vi "save as.vi"(8 "error in":errorcluster, 11 "state in":T1) -> (0 "error out":errorcluster, 1 "canceled?":bool, 3 "state out":T1)   [LabVIEW 2013, in "RT Temperature Controller.lvlib"]
uses:
  RT Temperature Controller.lvlib
  Controls/StateCluster.ctl
  <vilib>/NI/Tag Bus Data Framework/Configuration Editor/Classes/SystemConfigRepo/SystemConfigRepo.lvclass
  <vilib>/CEF_TreeControl/Node/NodeRef.ctl
  <vilib>/CEF_TreeControl/Node/NISE_CEF_Node.lvclass
  <vilib>/CEF_TreeControl/Node/UserEventRef.ctl
  <vilib>/CEF_TreeControl/Controls/EventCluster.ctl
  SplashScreen/splash screen.ctl
  SplashScreen/notifier data.ctl
  <vilib>/CEF_TreeControl/NISE_CEF_TreeControl.lvlib
  SplashScreen/splash screen.lvlib
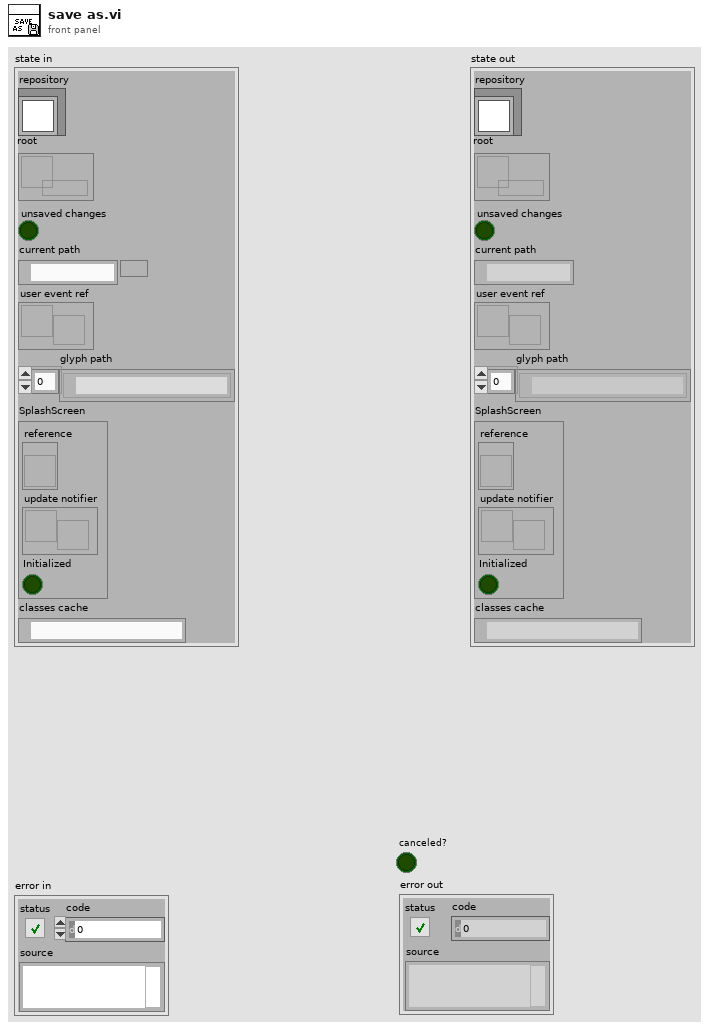
[diagram p1: front panel]
types:
  T1 = typedef "RT Temperature Controller.lvlib/StateCluster.ctl" = cluster{"repository":refnum<class "SystemConfigRepo.lvclass">, "root":T2, "unsaved changes":bool, "current path":path, "user event ref":T3, "glyph path":path[], "SplashScreen":T4, "classes cache":path}
  T2 = typedef "NISE_CEF_Node.lvclass/NodeRef.ctl" = refnum<data-value>
  T3 = typedef "NISE_CEF_Node.lvclass/UserEventRef.ctl" = refnum<user-event>
  T4 = typedef "RT Temperature Controller.lvlib/splash screen.lvlib/splash screen.ctl" = cluster{"reference":refnum<vi>, "update notifier":refnum<notifier>, "Initialized":bool}
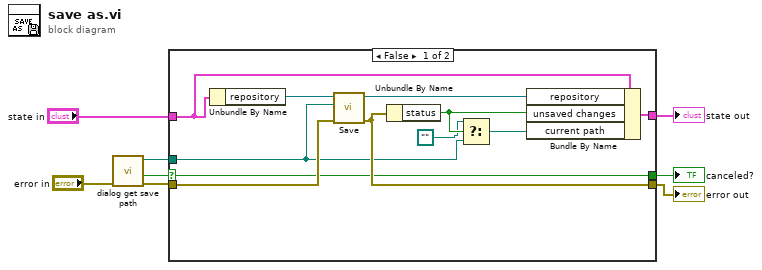
[diagram p0: block diagram]
diagram:
  n1 = call "dialog get save path.vi"("error in"="error in") -> ("error out"=w4:errorcluster, "cancelled"=w2:bool, "selected path"=w3:path)  [unwired: 8 in]
  n2 = case shown="False" w2 {
    selector: w2 -> [w13 w21]
    tunnel: "state in" -> [w17 w22]
    tunnel: w4 -> [w16 w20]
    tunnel: [w15 w20] -> w7
    tunnel: [w14 w22] -> w6
    tunnel: w3 -> [w11 _]
    tunnel: [w13 w21] -> w1
    frame False {
      n3 = Unbundle By Name(w17) -> ("repository"=w19:refnum<class "SystemConfigRepo.lvclass">)
      n4 = call-dynamic "Save.vi"("error in"=w16, "file path"=w11, "SystemConfigRepo in"=w19) -> ("error out"=w15:errorcluster, "SystemConfigRepo out"=w18:refnum<class "SystemConfigRepo.lvclass">)  [unwired: 7 in]
      n5 = Unbundle By Name(w15) -> ("status"=w12:bool)
      n6 = Select(t=path "", s=w12, f=w11) -> (s? t:f=w10:path)
      n7 = Bundle By Name(cluster=w17, "repository"=w18, "unsaved changes"=w12, "current path"=w10) -> (w14:T1)
    }
    frame True {
    }
  }
  "state out" <- w6
  "error out" <- w7
  "canceled?" <- w1
